vi "Get Display String.vi"(8 "error in":errorcluster, 11 "test\nresults in":refnum<class "Test Results Base Class.lvclass">) -> (0 "error out":errorcluster, 2 "display string":string, 3 "test results out":refnum<class "Test Results Base Class.lvclass">)   [LabVIEW 2020, in "Test Results Base Class.lvclass"]
doc: "This VI is an example of a protected member VI of a LabVIEW class. Only VIs within the same class or a descendant class can call this VI. This is also an example of a dynamic member VI."
uses:
  Test Results Base Class.lvclass
panel:
  # "This VI is an example of a dynamic member VI. It has protected access scope\nso that VIs outside of its class hierarchy cannot call it."
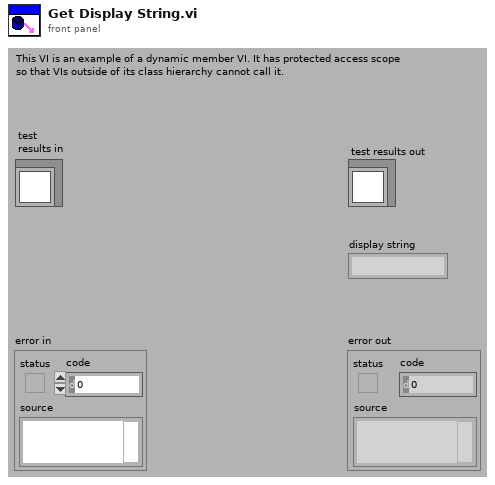
[diagram p1: front panel]
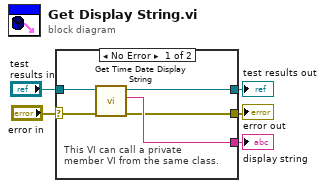
[diagram p0: block diagram]
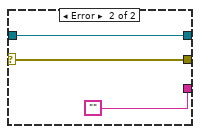
[diagram p2: hidden frame]
diagram:
  n1 = case shown="No Error" "error in" {
    selector: "error in" -> [w7 w12]
    tunnel: [w6 w13] -> w4
    tunnel: "test\nresults in" -> [w10 w13]
    tunnel: [w9 "" ("Empty String Constant")] -> w3
    tunnel: [w8 w12] -> w1
    frame No Error {
      # "This VI can call a private \nmember VI from the same class."
      n2 = call "Get Time Date Display String.vi"("error in \n(no error)"=w7, "test\n results in"=w10) -> ("error out"=w8:errorcluster, "concatenated string"=w9:string, "test results out"=w6:refnum<class "Test Results Base Class.lvclass">)  [unwired: 7 in]
    }
    frame Error {
    }
  }
  "error out" <- w1
  "test results out" <- w4
  "display string" <- w3
